vi "fromXMLNative.vi"(8 "error in (no error)":errorcluster, 10 "scriptEventListXML":refnum<k20>, 11 "ScriptEventList in":refnum<class "ScriptEventList.lvclass">) -> (0 "error out":errorcluster, 3 "ScriptEventList out":refnum<class "ScriptEventList.lvclass">)   [LabVIEW 2009, in "Tools.lvlib" / "Scripting.lvlib" / "ScriptEventList.lvclass"]
uses:
  ScriptEventList.lvclass
  <vilib>/xml/Close Reference(Node).vi
  ScriptEventList.lvclass/ScriptEventList.ctl
  <vilib>/xml/NI_XML.lvlib
  ScriptEvent.lvclass
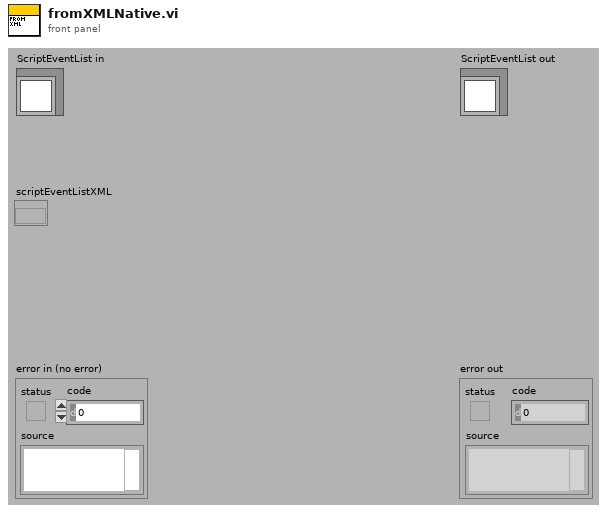
[diagram p1: front panel]
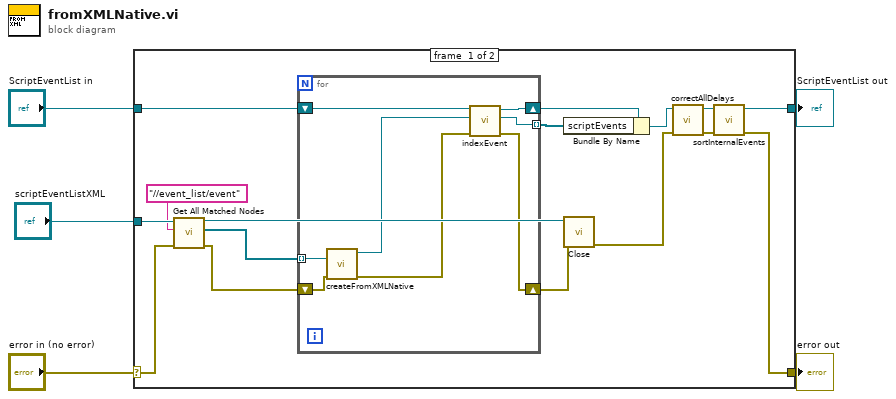
[diagram p0: block diagram]
diagram:
  n1 = case shown="No Error" "error in (no error)" {
    selector: "error in (no error)" -> [w16 w31]
    tunnel: [w7 w31] -> w4
    tunnel: [w8 w30] -> w2
    tunnel: "ScriptEventList in" -> [w15 w30]
    tunnel: "scriptEventListXML" -> [w21 _]
    frame #0 {
      n2 = call <vilib>:"Get All Matched Nodes.vi"("error in (no error)"=w16, "XPath expression"="//event_list/event", "node in"=w21) -> ("error out"=w17:errorcluster, "node result array"=w19:refnum<k20>[], "node out"=w18:refnum<k20>)  [unwired: 6 in]
      n3 = for {
        tunnel: w19 -> [w26] mode=indexing
        shift-right: [w28] -> w12
        shift-left: w15 -> [w29]
        shift-right: [w27] -> w14
        shift-left: w17 -> [w25]
        tunnel: [w22] -> w13 mode=indexing
        n4 = call "createFromXMLNative.vi"("error in (no error)"=w25, "scriptEventXML"=w26) -> ("error out"=w23:errorcluster, "ScriptEvent out"=w24:refnum<class "ScriptEvent.lvclass">)  [unwired: 8 in]
        n5 = call "indexEvent.vi"("error in (no error)"=w23, "ScriptEvent"=w24, "ScriptEventList in"=w29) -> ("error out"=w27:errorcluster, "ScriptEvent out"=w22:refnum<class "ScriptEvent.lvclass">, "ScriptEventList out"=w28:refnum<class "ScriptEventList.lvclass">)  [unwired: 5 in, 1 out]
      }
      n6 = Bundle By Name(cluster=w12, "scriptEvents"=w13) -> (w9:refnum<class "ScriptEventList.lvclass">)
      n7 = call-poly <vilib>:"Close.vi"("error in (no error)"=w14, "node"=w18) -> ("error out"=w6:errorcluster)  [unwired: 7 in]
      n8 = call "correctAllDelays.vi"("error in (no error)"=w6, "ScriptEventList in"=w9) -> ("error out"=w10:errorcluster, "ScriptEventList out"=w11:refnum<class "ScriptEventList.lvclass">)  [unwired: 8 in]
      n9 = call "sortInternalEvents.vi"("error in (no error)"=w10, "ScriptEventList in"=w11) -> ("error out"=w7:errorcluster, "ScriptEventList out"=w8:refnum<class "ScriptEventList.lvclass">)  [unwired: 8 in]
    }
    frame #1 {
    }
  }
  "error out" <- w4
  "ScriptEventList out" <- w2
